vi "Set Alpha.vi"(8 "error in (no error)":errorcluster, 10 "alpha":i32 min=0 max=255, 11 "Color in":refnum<class "Color.lvclass">) -> (0 "error out":errorcluster, 3 "Color out":refnum<class "Color.lvclass">)   [LabVIEW 2013, in "DataGrid.lvlib" / "Color.lvclass"]
doc: "Sets the alpha transparency of the Color class from 0 to 255. 255 is fully opaque and 0 is fully transparent."
uses:
  Color.lvclass
  System.Drawing
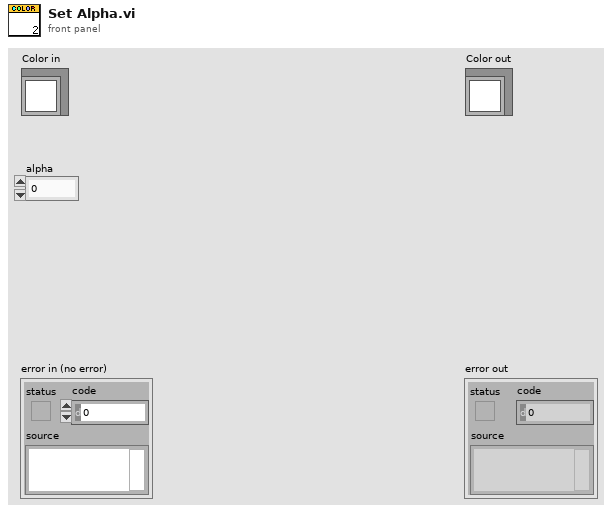
[diagram p1: front panel]
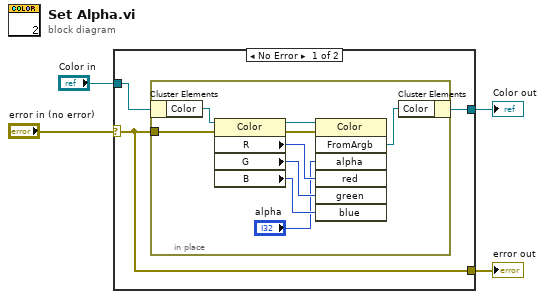
[diagram p0: block diagram]
diagram:
  n1 = case shown="No Error" "error in (no error)" {
    selector: "error in (no error)" -> [w7 w18]
    tunnel: [w7 w18] -> w3
    tunnel: [w5 w17] -> w1
    tunnel: "Color in" -> [w6 w17]
    frame No Error {
      n2 = in-place {
        in-place-border: w7 -> [w9]
        n3 = in-place-cluster #1(w6) -> ("Color"=w10:refnum<k24>)
        n4 = property class="Color"(reference=w10, error in=w9) -> (reference out=w16:refnum<k24>, error out=w15:errorcluster, "R"=w14:u8, "G"=w13:u8, "B"=w12:u8)
        n5 = invoke class="Color" method="FromArgb"(reference=w16, error in=w15, "alpha"="alpha", "red"=w14, "green"=w13, "blue"=w12) -> ("FromArgb"=w8:refnum<k24>)  [unwired: 1 in, 6 out]
        n6 = in-place-cluster #1("Color"=w8) -> (w5:refnum<class "Color.lvclass">)
      }
    }
    frame Error {
    }
  }
  "error out" <- w3
  "Color out" <- w1
